vi "Close Tab Button - Label--Const.vi"() -> (3 "Close Tab Control Label":string)   [LabVIEW 2017, in "DTacq Plot Display Library.lvlib"]
uses:
  DTacq Plot Display Library.lvlib
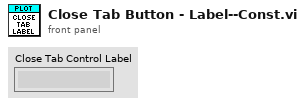
[diagram p1: front panel]
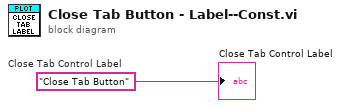
[diagram p0: block diagram]
diagram:
  w1 = "Close Tab Button"  # Close Tab Control Label
  "Close Tab Control Label" <- w1
